vi "Measurement.vi"(8 "error in (no error)":errorcluster, 9 "Grandeza":string, 10 "Multiplicador":dbl, 11 "189 in":refnum<class "189.lvclass">) -> (0 "error out":errorcluster, 2 "Measurement":dbl, 3 "189 out":refnum<class "189.lvclass">)   [LabVIEW 2015, in "189.lvclass"]
doc: "VI used to measure Value using the multimeter"
uses:
  189.lvclass
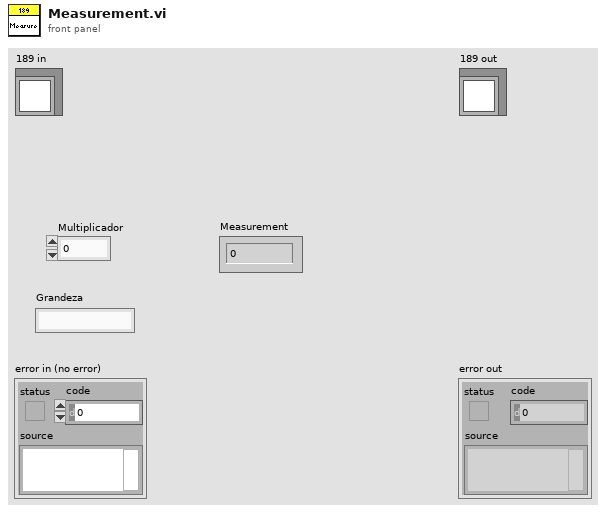
[diagram p1: front panel]
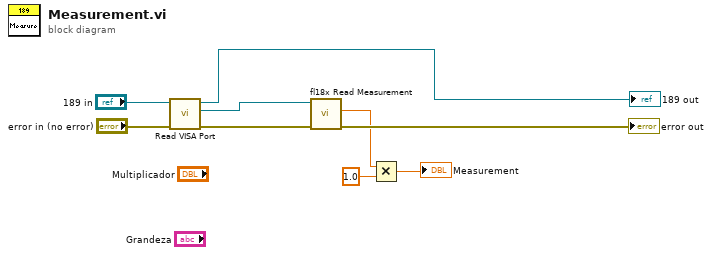
[diagram p0: block diagram]
diagram:
  n1 = call-dynamic "Read VISA Port.vi"("error in (no error)"="error in (no error)", "Device in"="189 in") -> ("error out"=w6:errorcluster, "VISA Port"=w7:refnum<visa-resource-name>, "Device out"=→"189 out":refnum<class "189.lvclass">)  [unwired: 7 in]
  n2 = call <instrlib>:"fl18x Read Measurement.vi"("error in (no error)"=w6, "VISA session"=w7) -> ("error out"=→"error out":errorcluster, "Measurement"=w3:dbl)  [unwired: 5 in, 3 out]
  n3 = Multiply(x=w3, y=1.0) -> (x*y=→"Measurement":dbl)
